vi "NI5112.i attribute.vi"(0 "VI Refnum":refnum<vi>, 2 "CLASS.i attribute":T1, 3 "Action":T2(ring), 5 "error in (no error)":errorcluster) -> (14 "VI Refnum out":refnum<vi>, 16 "CLASS.i attribute out":T1, 19 "error out":errorcluster)   [LabVIEW 2014, in "NI5112.lvlib"]
doc: "This is a so-called functional global variable. It manages the access to a global variable in a thread-safe way. \n\nHere the attribute data of all instances of THIS class are stored. This is done for performance reasons.\n\nLicense Agreement for this software:\n\nCopyright (C)\nGesellschaft für Schwerionenforschung, GSI\nPlanckstr. 1\n64291 Darmstadt\nGermany\n\nContact: D.Beck@gsi.de \n\nThis program is free software; you can redistribute it and/or modify it under the terms of the GNU General Public License as published by the Free Software Foundation; either version 2 of the license, or (at your option) any later version.\n\nThis program is distributed in the hope that it will be useful, but WITHOUT ANY WARRANTY; without even the implied warranty of MERCHANTABILITY or FITNESS FOR A PARTICULAR PURPOSE. See the GNU General License for more details (http://www.gnu.org).\n\nGesellschaft für Schwerionenforschung, GSI\nPlanckstr. 1, 64291 Darmstadt, Germany\nFor all questions and ideas contact: M.Richter@gsi.de, H.Brand@gsi.de or D.Beck@gsi.de.\nLast update: 17-JUN-2004"
uses:
  NI5112.lvlib
  NI5112.i attribute.ctl
  CSCore/CSSystem/CoreDefs/CoreDefs.error_type.ctl
  CSCore/CSSystem/CoreLib/CoreLib.lvlib
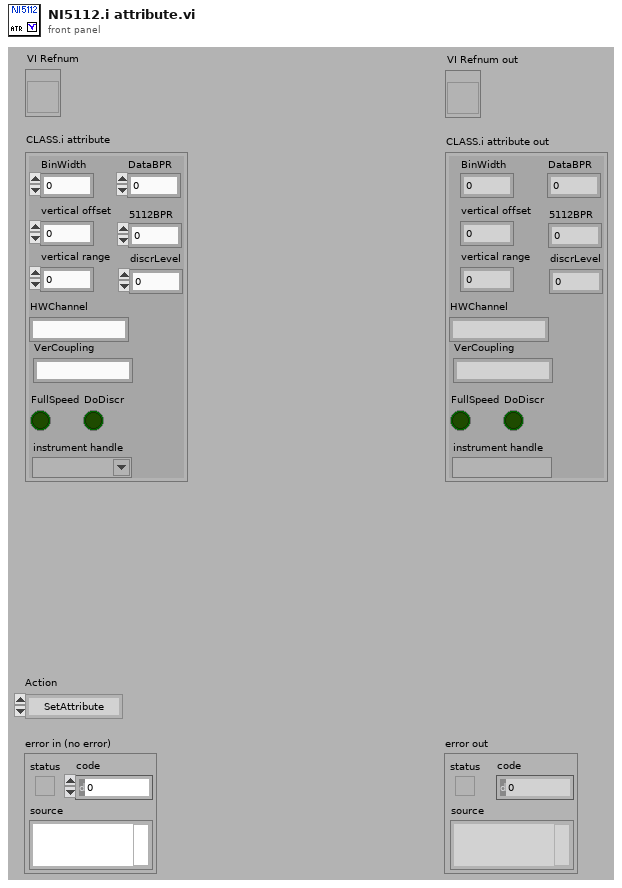
[diagram p1: front panel]
types:
  T1 = typedef "NI5112.lvlib/NI5112.i attribute.ctl" = cluster{"HWChannel":string, "instrument handle":refnum<k15>, "BinWidth":dbl, "vertical offset":dbl, "vertical range":dbl, "DataBPR":i32, "5112BPR":i32, "FullSpeed":bool, "discrLevel":dbl, "DoDiscr":bool, "VerCoupling":string}
  T2 = enum16{"SetAttribute", "GetAttribute", "CreateAttribute", "DestroyAttribute", "DestroyAllAtributes"}
  T3 = typedef "CoreDefs.error_type.ctl" = enum16{"no error", "can't load process", "can't unload process", "process does not exist", "can't install process", "can't remove process", "unknown function", "time out", "can't execute function", "duplicate queue name", "super not found", "caller queue invalid", "can't ping process", "unknown error", "VISA Error", "VISA timeout", "GPIB timeout", "GPIB error", "communication error", "data type mismatch", "can't read data from OPC server", "can't write data to OPC server", "OET error", "function not implemented", "process already exists", "invalid Shared Variable name", "error writing Shared Variable", "error reading Shared Variable", "invalid client name", "corrupt database", "unknown class", "call not authorized", "parameter out of range", "OET timeout: can't get data to modify", "invalid queue name", "requested operation incompatible with current state", "event undefined", "event disabled", "state undefined", "caller is not a friend", "EventBuilder: bad eventID", "EventBuilder: no DAQ devices", "a thread must not stop itself", "UNUSED ELEMENT4", "DiscArchiver: eventData incomplete", "DiscArchiver: eventData does not belong to run", "DiscArchiver: can't open file", "DiscArchiver: can't write to file", "DiscArchiver: available disc space low", "can't acquire semaphore", "error reading data from database", "notifier object is not existing", "can't register process", "can't unregister process", "illegal event type", "object disabled", "object already exists", "can't change state", "Instrument not found", "no connection to remote node", "invalid reference", "N/A", "UNUSED ELEMENT 1", "element not found", "illegal TCP/IP connection detected", "object does not exist", "invalid access ID", "unknown CS system", "invalid privilige", "unsupported data type", "unsupported server type", "IO server already exists", "Shared Variable already exists"}
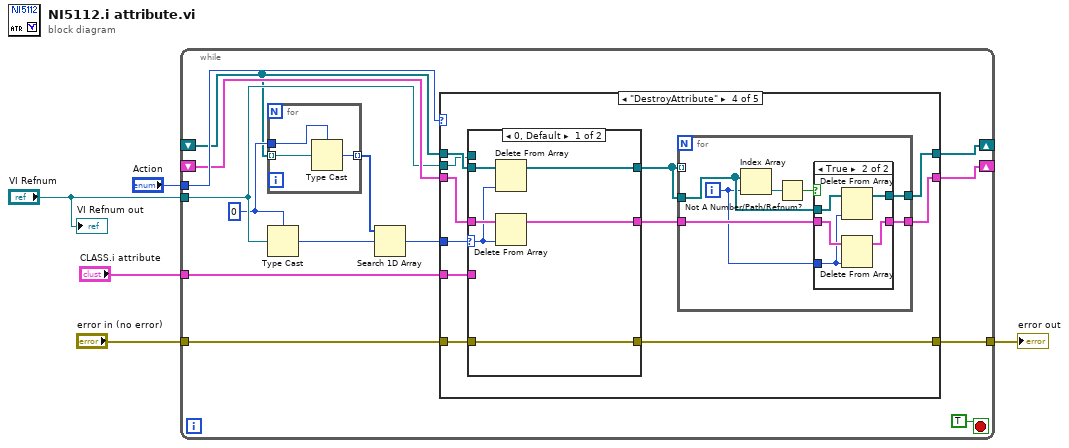
[diagram p0: block diagram]
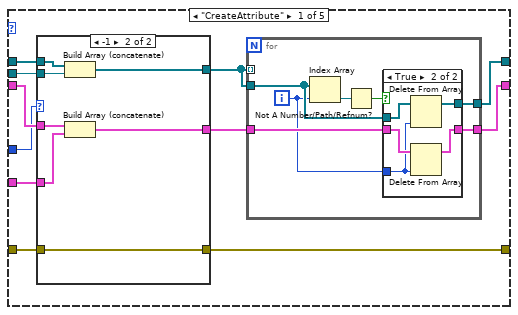
[diagram p2: hidden frame]
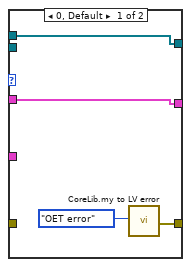
[diagram p4: hidden frame]
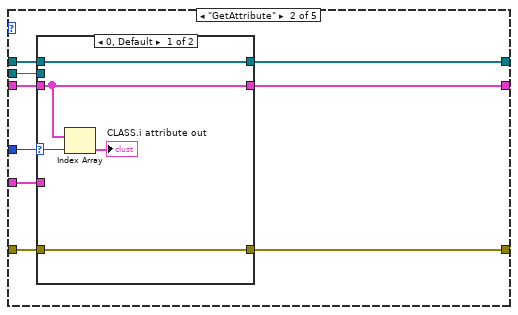
[diagram p5: hidden frame]
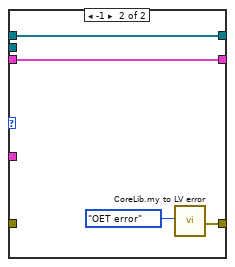
[diagram p6: hidden frame]
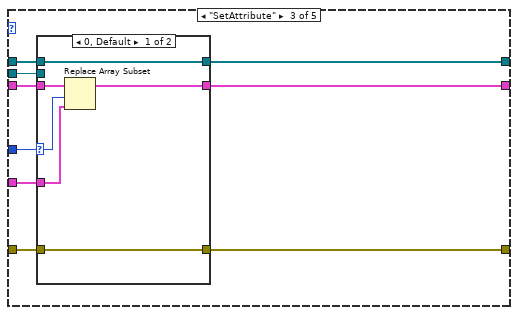
[diagram p7: hidden frame]
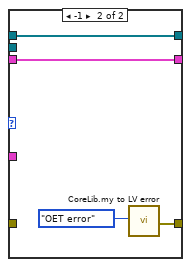
[diagram p8: hidden frame]
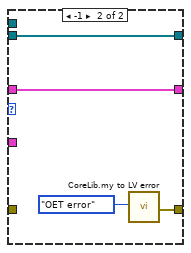
[diagram p10: hidden frame]
diagram:
  n1 = while {
    shift-right: [w13] -> _
    shift-left: _ -> [w14]
    tunnel: "Action" -> [w18]
    shift-right: [w15] -> _
    shift-left: _ -> [w6]
    tunnel: "error in (no error)" -> [w17]
    tunnel: [w16] -> w3
    tunnel: "CLASS.i attribute" -> [w12]
    tunnel: "VI Refnum" -> [w9]
    stop <- TRUE stop-if-true
    w8 = 0
    n2 = for {
      tunnel: w8 -> [w22]
      tunnel: [w21] -> w7 mode=indexing
      tunnel: w6 -> [w20] mode=indexing
      n3 = Type Cast(type=w22, x=w20) -> (*(type *) &x=w21:i32)
    }
    n4 = Type Cast(type=w8, x=w9) -> (*(type *) &x=w10:i32)
    n5 = Search 1D Array(1D array=w7, element=w10) -> (index of element=w11:i32)  [unwired: 1 in]
    n6 = case shown="\"DestroyAttribute\"" w18 {
      tunnel: w6 -> [w31 w65 w83 w104 _]
      tunnel: w9 -> [w30 w63 w81 w103 _]
      tunnel: w17 -> [w33 w67 w85 w106 w131]
      tunnel: [w32 w66 w84 w105 w131] -> w16
      tunnel: [w26 w64 w82 w98 _] -> w15
      tunnel: w14 -> [w29 w62 w80 w102 _]
      tunnel: [w24 w61 w79 w97 _] -> w13
      tunnel: w12 -> [w28 w60 w78 w101 _]
      tunnel: w11 -> [w27 w59 w77 w100 _]
      frame "CreateAttribute" {
        n7 = case shown="-1" w27 {
          tunnel: w33 -> [_ w58]
          tunnel: [w50 w58] -> w32
          tunnel: w31 -> [w49 w57]
          tunnel: [w49 w56] -> w23
          tunnel: w30 -> [_ w55]
          tunnel: w29 -> [w48 w54]
          tunnel: [w48 w53] -> w25
          tunnel: w28 -> [_ w52]
          frame 0, Default {
            n8 = call "CoreLib.my to LV error.vi"("ErrorTypes"=CoreDefs.error_type."OET error") -> ("myErrorCluster"=w50:errorcluster)  [unwired: 17 in, 1 out]
          }
          frame -1 {
            n9 = Build Array (concatenate)(w57, w55) -> (w56:refnum<vi>[])
            n10 = Build Array (concatenate)(w54, w52) -> (w53:T1[])
          }
        }
        n11 = for {
          tunnel: w23 -> [w36]
          tunnel: [w35] -> w26
          tunnel: [w40] -> w24
          tunnel: w25 -> [w39]
          tunnel: w23 -> [_] mode=indexing
          i -> [w34]
          n12 = Index Array(array=w36, index=w34) -> (element=w37:refnum<vi>)
          n13 = Not A Number/Path/Refnum?(number/path/refnum=w37) -> (NaN/Path/Refnum?=w38:bool)
          n14 = case shown="True" w38 {
            tunnel: [w42 w47] -> w40
            tunnel: w39 -> [w42 w46]
            tunnel: [w41 w44] -> w35
            tunnel: w36 -> [w41 w45]
            tunnel: w34 -> [_ w43]
            frame False {
            }
            frame True {
              n15 = Delete From Array(array=w45, index=w43) -> (array with subset deleted=w44:refnum<vi>[])  [unwired: 1 in, 1 out]
              n16 = Delete From Array(array=w46, index=w43) -> (array with subset deleted=w47:T1[])  [unwired: 1 in, 1 out]
            }
          }
        }
      }
      frame "GetAttribute" {
        n17 = case shown="0, Default" w59 {
          selector: w59 -> [w70 _]
          tunnel: w67 -> [w72 _]
          tunnel: [w72 w75] -> w66
          tunnel: w65 -> [w71 w74]
          tunnel: [w71 w74] -> w64
          tunnel: w63 -> [_ _]
          tunnel: w62 -> [w69 w73]
          tunnel: [w69 w73] -> w61
          tunnel: w60 -> [_ _]
          frame 0, Default {
            n18 = Index Array(array=w69, index=w70) -> (element=→"CLASS.i attribute out":T1)
          }
          frame -1 {
            n19 = call "CoreLib.my to LV error.vi"("ErrorTypes"=CoreDefs.error_type."OET error") -> ("myErrorCluster"=w75:errorcluster)  [unwired: 17 in, 1 out]
          }
        }
      }
      frame "SetAttribute" {
        n20 = case shown="0, Default" w77 {
          selector: w77 -> [w87 _]
          tunnel: w85 -> [w91 _]
          tunnel: [w91 w94] -> w84
          tunnel: w83 -> [w90 w93]
          tunnel: [w90 w93] -> w82
          tunnel: w81 -> [_ _]
          tunnel: w80 -> [w89 w92]
          tunnel: [w88 w92] -> w79
          tunnel: w78 -> [w86 _]
          frame 0, Default {
            n21 = Replace Array Subset(array=w89, new element=w86, index=w87) -> (w88:T1[])
          }
          frame -1 {
            n22 = call "CoreLib.my to LV error.vi"("ErrorTypes"=CoreDefs.error_type."OET error") -> ("myErrorCluster"=w94:errorcluster)  [unwired: 17 in, 1 out]
          }
        }
      }
      frame "DestroyAttribute" {
        n23 = case shown="0, Default" w100 {
          selector: w100 -> [w122 _]
          tunnel: w106 -> [w126 _]
          tunnel: [w126 w129] -> w105
          tunnel: w104 -> [w125 w128]
          tunnel: [w124 w128] -> w96
          tunnel: w103 -> [_ _]
          tunnel: w102 -> [w123 w127]
          tunnel: [w121 w127] -> w99
          tunnel: w101 -> [_ _]
          frame 0, Default {
            n24 = Delete From Array(array=w125, index=w122) -> (array with subset deleted=w124:refnum<vi>[])  [unwired: 1 in, 1 out]
            n25 = Delete From Array(array=w123, index=w122) -> (array with subset deleted=w121:T1[])  [unwired: 1 in, 1 out]
          }
          frame -1 {
            n26 = call "CoreLib.my to LV error.vi"("ErrorTypes"=CoreDefs.error_type."OET error") -> ("myErrorCluster"=w129:errorcluster)  [unwired: 17 in, 1 out]
          }
        }
        n27 = for {
          tunnel: w96 -> [w109]
          tunnel: [w108] -> w98
          tunnel: [w113] -> w97
          tunnel: w99 -> [w112]
          tunnel: w96 -> [_] mode=indexing
          i -> [w107]
          n28 = Index Array(array=w109, index=w107) -> (element=w110:refnum<vi>)
          n29 = Not A Number/Path/Refnum?(number/path/refnum=w110) -> (NaN/Path/Refnum?=w111:bool)
          n30 = case shown="True" w111 {
            tunnel: [w115 w120] -> w113
            tunnel: w112 -> [w115 w119]
            tunnel: [w114 w117] -> w108
            tunnel: w109 -> [w114 w118]
            tunnel: w107 -> [_ w116]
            frame False {
            }
            frame True {
              n31 = Delete From Array(array=w118, index=w116) -> (array with subset deleted=w117:refnum<vi>[])  [unwired: 1 in, 1 out]
              n32 = Delete From Array(array=w119, index=w116) -> (array with subset deleted=w120:T1[])  [unwired: 1 in, 1 out]
            }
          }
        }
      }
      frame "DestroyAllAtributes" {
      }
    }
  }
  "error out" <- w3
  "VI Refnum out" <- "VI Refnum"
